vi "solar_voy EnQ (ID).vi"(7 "Setup":T1, 8 "error in (no error)":errorcluster, 9 "ID":u16, 10 "TCP Data":string, 11 "Voyager Refnum in":T2) -> (0 "error out":errorcluster, 3 "Voyager Refnum out":T2)   [LabVIEW 2018]
doc: "This unpacks the TCP message and enqueues the message to the target. The 'HDR_GUID' is added to the message data variant attibutes."
uses:
  solar_voy_ctl Voyager Refnum.ctl
  solar_voy_ctl Port Setup.ctl
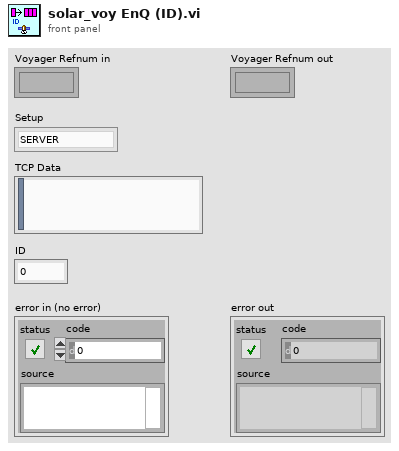
[diagram p1: front panel]
types:
  T1 = typedef "solar_voy_ctl Port Setup.ctl" = enum8{"SERVER", "CLIENT", "SERVER_CMD", "SERVER_TLM"}
  T2 = typedef "solar_voy_ctl Voyager Refnum.ctl" = refnum<k1>
  T3 = typedef "solar_voy_def_ctl HDR.ctl" = cluster{"ITEMS":T4[], "LENGTH_NAME":string, "LENGTH_VALUE_OFFSET":i32, "ID_NAME":string, "ENDIAN":enum8{"BIG", "LITTLE"}, "GUID_NAME":string, "DEFAULT_TARGET":string, "DEFAULT_PACKET":string, "DEFAULT_ERROR":string}
  T4 = typedef "solar_voy_def_ctl ITEM.ctl" = cluster{"NAME":string, "OFFSET":i32, "SIZE":i32, "TYPE":T5, "EACH_SIZE":i32, "LVTYPE":T6, "MIN":dbl, "MAX":dbl, "DEFAULT":string, "DESC":string, "ID":bool, "MODIFIERS":variant, "last_value":variant}
  T5 = typedef "solar_voy_def_ctl ITEM TYPE.ctl" = enum8{"BLOCK", "INT", "UINT", "FLOAT", "STRING"}
  T6 = typedef "solar_type Item Type.ctl" = enum16{"NULL", "UNKNOWN", "CLUSTER", "I8", "I16", "I32", "I64", "U8", "U16", "U32", "U64", "U8_ENUM", "U16_ENUM", "U32_ENUM", "SGL", "DBL", "BOOLEAN", "STRING", "PATH", "VISA", "TAG", "TIME", "I8_1D", "I16_1D", "I32_1D", "I64_1D", "U8_1D", "U16_1D", "U32_1D", "U64_1D", "U8_ENUM_1D", "U16_ENUM_1D", "U32_ENUM_1D", "SGL_1D", "DBL_1D", "BOOLEAN_1D", "STRING_1D", "PATH_1D", "VISA_1D", "TAG_1D", "TIME_1D", "I8_2D", "I16_2D", "I32_2D", "I64_2D", "U8_2D", "U16_2D", "U32_2D", "U64_2D", "U8_ENUM_2D", "U16_ENUM_2D", "U32_ENUM_2D", "SGL_2D", "DBL_2D", "BOOLEAN_2D", "STRING_2D", "PATH_2D", "VISA_2D", "TAG_2D", "TIME_2D"}
  T7 = typedef "solar_voy_def_ctl PACKET.ctl" = cluster{"PACKET_ID":T8, "ENDIAN":enum8{"BIG", "LITTLE"}, "DESC":string, "HZRD":bool, "ITEMS":T4[], "NoExport":bool, "last_time":timestamp, "last_count":u32, "last_data":string}
  T8 = typedef "solar_voy_def_ctl PACKET_ID.ctl" = cluster{"ID":u16, "CMD":enum8{"CMD", "TLM"}, "TARGET":string, "PACKET":string}
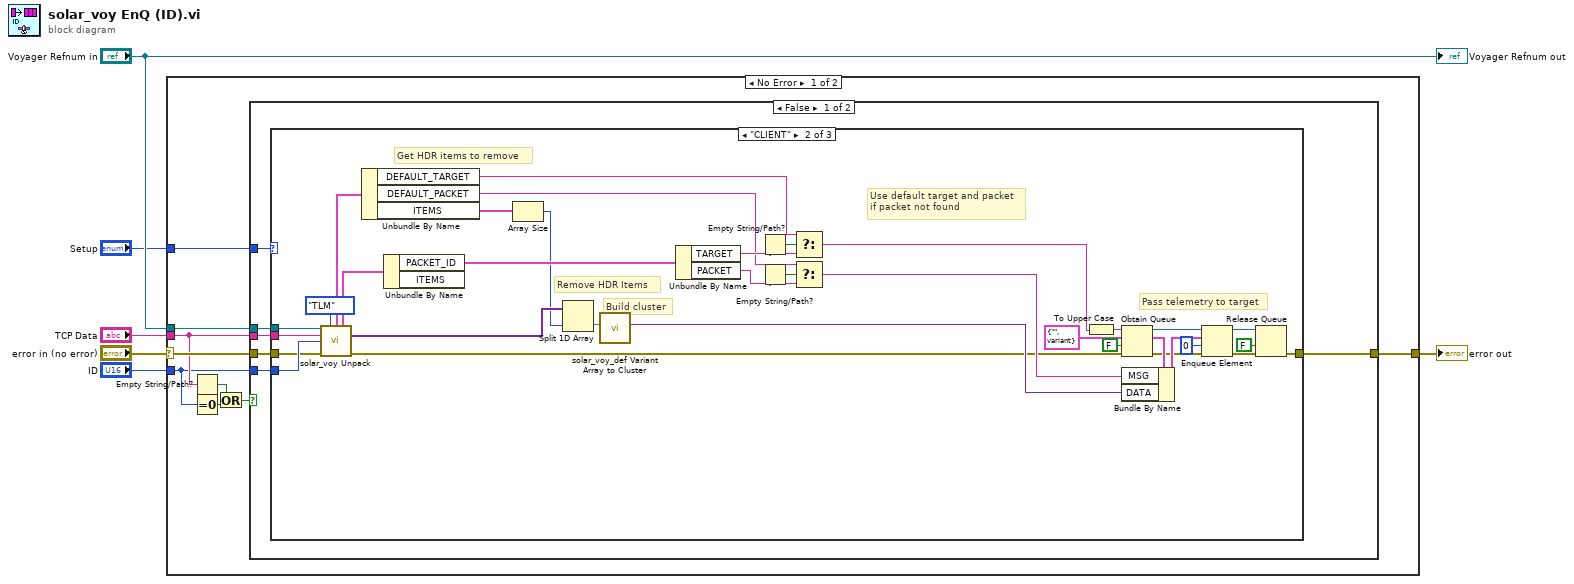
[diagram p0: block diagram]
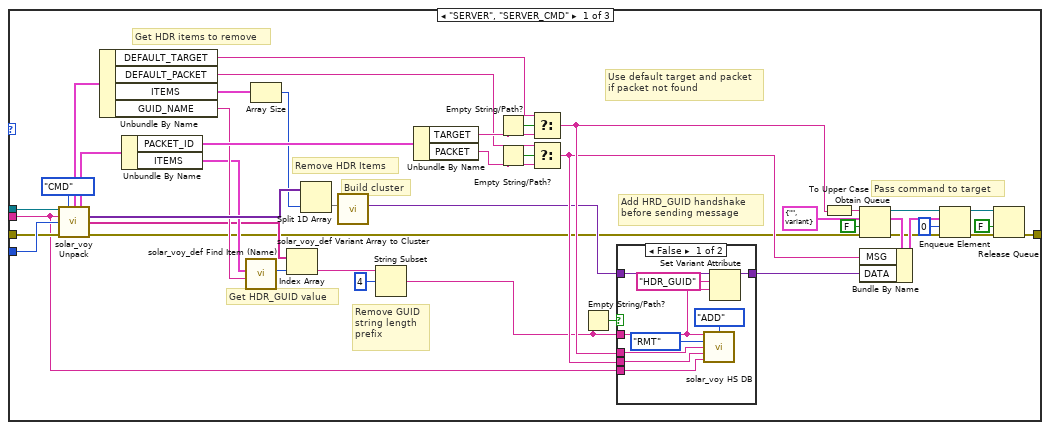
[diagram p2: hidden frame]
diagram:
  n1 = case shown="No Error" "error in (no error)" {
    selector: "error in (no error)" -> [w14 w109]
    tunnel: [w15 w109] -> w6
    tunnel: "Voyager Refnum in" -> [w12 _]
    tunnel: "TCP Data" -> [w11 _]
    tunnel: "ID" -> [w10 _]
    tunnel: "Setup" -> [w13 _]
    frame No Error {
      n2 = Empty String/Path?(string/path=w11) -> (empty?=w8:bool)
      n3 = Equal To 0?(x=w10) -> (x = 0?=w9:bool)
      n4 = Or(x=w8, y=w9) -> (x .or. y?=w7:bool)
      n5 = case shown="False" w7 {
        tunnel: [w21 w108] -> w15
        tunnel: w14 -> [w18 w108]
        tunnel: w10 -> [w19 _]
        tunnel: w13 -> [w16 _]
        tunnel: w11 -> [w17 _]
        tunnel: w12 -> [w20 _]
        frame False {
          n6 = case shown="\"CLIENT\"" w16 {
            tunnel: [w63 w106 w107] -> w21
            tunnel: w20 -> [w45 w88 _]
            tunnel: w19 -> [w44 w87 _]
            tunnel: w18 -> [w43 w86 w107]
            tunnel: w17 -> [w42 w85 _]
            frame "SERVER", "SERVER_CMD" {
              w60 = cluster{"MSG":string, "DATA":variant} {"MSG"="", "DATA"=variant} ("MSG")
              # "Remove GUID\nstring length\nprefix"
              # "Get HDR_GUID value"
              # "Get HDR items to remove"
              # "Build cluster"
              # "Remove HDR Items"
              # "Add HRD_GUID handshake\nbefore sending message"
              # "Use default target and packet\nif packet not found"
              # "Pass command to target"
              n7 = call "solar_voy Unpack.vi"("Voyager Refnum in"=w45, "CMD"=enum8{"CMD", "TLM"}."CMD", "TCP Data"=w42, "ID"=w44, "error in (no error)"=w43) -> ("HDR"=w37:T3, "PACKET"=w38:T7, "Item Values"=w36:variant[], "Item Values (LV Flattened Value)"=w30:string[], "error out"=w26:errorcluster)  [unwired: 4 in, 2 out]
              n8 = Unbundle By Name(w37) -> ("DEFAULT_TARGET"=w47:string, "DEFAULT_PACKET"=w46:string, "ITEMS"=w33:T4[], "GUID_NAME"=w34:string)
              n9 = Unbundle By Name(w38) -> ("PACKET_ID"=w49:T8, "ITEMS"=w32:T4[])
              n10 = call "solar_voy_def Find Item (Name).vi"("ITEM_NAME"=w34, "ITEMS"=w32) -> ("Index"=w31:i32)  [unwired: 9 in]
              n11 = Array Size(array=w33) -> (size(s)=w35:i32)
              n12 = Index Array(array=w30, index=w31) -> (element=w25:string)
              n13 = Split 1D Array(array=w36, index=w35) -> (second subarray=w39:variant[])  [unwired: 1 out]
              n14 = call "solar_voy_def Variant Array to Cluster.vi"("Variant Elements"=w39) -> ("Cluster Variant"=w28:variant)  [unwired: 10 in]
              n15 = String Subset(string=w25, offset (0)=4) -> (substring=w24:string)  [unwired: 1 in]
              n16 = Unbundle By Name(w49) -> ("TARGET"=w52:string, "PACKET"=w50:string)
              n17 = Empty String/Path?(string/path=w52) -> (empty?=w53:bool)
              n18 = Empty String/Path?(string/path=w50) -> (empty?=w51:bool)
              n19 = Select(t=w47, s=w53, f=w52) -> (s? t:f=w41:string)
              n20 = Select(t=w46, s=w51, f=w50) -> (s? t:f=w40:string)
              n21 = Empty String/Path?(string/path=w24) -> (empty?=w29:bool)
              n22 = case shown="False" w29 {
                tunnel: w42 -> [w72 _]
                tunnel: w41 -> [w71 _]
                tunnel: w40 -> [w70 _]
                tunnel: w24 -> [w64 _]
                tunnel: w28 -> [w67 w73]
                tunnel: [w66 w73] -> w27
                frame False {
                  n23 = call "solar_voy HS DB.vi"("HDR_GUID"=w64, "Action"=enum8{"DELETE", "ADD", "CLEAR"}."ADD", "ORIGIN in"=enum8{"RMT", "LCL"}."RMT" ("HS_ORIGIN in"), "TARGET in"=w71, "PACKET in"=w70, "DATA in"=w72) -> ()  [unwired: 5 in, 5 out]
                  n24 = Set Variant Attribute(Variant=w67, name="HDR_GUID", value=w64) -> (Variant out=w66:variant)  [unwired: 1 in, 2 out]
                }
                frame True {
                  # "No HDR_GUID"
                }
              }
              n25 = To Upper Case(1:w41) -> (0:w48:string)
              n26 = Obtain Queue(name (unnamed)=w48, element data type=w60, create if not found? (T)=FALSE, error in (no error)=w26) -> (queue out=w54:refnum<queue>, error out=w59:errorcluster)  [unwired: 1 in, 1 out]
              n27 = Bundle By Name(cluster=w60, "MSG"=w40, "DATA"=w27) -> (w61:cluster{"MSG":string, "DATA":variant})
              n28 = Enqueue Element(queue=w54, element=w61, timeout in ms (-1)=0, error in (no error)=w59) -> (queue out=w57:refnum<queue>, error out=w58:errorcluster)  [unwired: 1 out]
              n29 = Release Queue(queue=w57, force destroy? (F)=FALSE, error in (no error)=w58) -> (error out=w63:errorcluster)  [unwired: 2 out]
            }
            frame "CLIENT" {
              w103 = cluster{"MSG":string, "DATA":variant} {"MSG"="", "DATA"=variant} ("MSG")
              # "Get HDR items to remove"
              # "Build cluster"
              # "Remove HDR Items"
              # "Use default target and packet\nif packet not found"
              # "Pass telemetry to target"
              n30 = call "solar_voy Unpack.vi"("Voyager Refnum in"=w88, "CMD"=enum8{"CMD", "TLM"}."TLM", "TCP Data"=w85, "ID"=w87, "error in (no error)"=w86) -> ("HDR"=w80:T3, "PACKET"=w81:T7, "Item Values"=w79:variant[], "error out"=w75:errorcluster)  [unwired: 4 in, 3 out]
              n31 = Unbundle By Name(w80) -> ("DEFAULT_TARGET"=w90:string, "DEFAULT_PACKET"=w89:string, "ITEMS"=w77:T4[])
              n32 = Unbundle By Name(w81) -> ("PACKET_ID"=w92:T8)  [unwired: 1 out]
              n33 = Array Size(array=w77) -> (size(s)=w78:i32)
              n34 = Split 1D Array(array=w79, index=w78) -> (second subarray=w82:variant[])  [unwired: 1 out]
              n35 = call "solar_voy_def Variant Array to Cluster.vi"("Variant Elements"=w82) -> ("Cluster Variant"=w76:variant)  [unwired: 10 in]
              n36 = Unbundle By Name(w92) -> ("TARGET"=w95:string, "PACKET"=w93:string)
              n37 = Empty String/Path?(string/path=w95) -> (empty?=w96:bool)
              n38 = Empty String/Path?(string/path=w93) -> (empty?=w94:bool)
              n39 = Select(t=w90, s=w96, f=w95) -> (s? t:f=w84:string)
              n40 = Select(t=w89, s=w94, f=w93) -> (s? t:f=w83:string)
              n41 = To Upper Case(1:w84) -> (0:w91:string)
              n42 = Obtain Queue(name (unnamed)=w91, element data type=w103, create if not found? (T)=FALSE, error in (no error)=w75) -> (queue out=w97:refnum<queue>, error out=w102:errorcluster)  [unwired: 1 in, 1 out]
              n43 = Bundle By Name(cluster=w103, "MSG"=w83, "DATA"=w76) -> (w104:cluster{"MSG":string, "DATA":variant})
              n44 = Enqueue Element(queue=w97, element=w104, timeout in ms (-1)=0, error in (no error)=w102) -> (queue out=w100:refnum<queue>, error out=w101:errorcluster)  [unwired: 1 out]
              n45 = Release Queue(queue=w100, force destroy? (F)=FALSE, error in (no error)=w101) -> (error out=w106:errorcluster)  [unwired: 2 out]
            }
            frame "SERVER_TLM" {
              # "Client should not send commands\n- Ignore any inbound messages"
            }
          }
        }
        frame True {
          # "Invalid ID or TCP Data\n- Do nothing"
        }
      }
    }
    frame Error {
    }
  }
  "error out" <- w6
  "Voyager Refnum out" <- "Voyager Refnum in"
